vi "BASE_Reporting.vi"(8 "error in (no error)":errorcluster) -> (0 "error out":errorcluster)   [LabVIEW 2017]
uses:
  <vilib>/Utility/miscctls.llb/LVRangeTypeDef.ctl
  <vilib>/Utility/miscctls.llb/LVRowAndColumnTypeDef.ctl
  <vilib>/Utility/miscctls.llb/LVRowAndColumnUnsignedTypeDef.ctl
  <vilib>/addons/database/Connection.llb/DB Tools Open Connec (Path).vi
  <vilib>/Utility/file.llb/Write Delimited Spreadsheet (string).vi
  <vilib>/addons/database/NI_Database_API.lvlib
panel:
  in  "Machine Selection":string(combo)="ALL STATION"
  in  "Horizontal Slider Control":dbl(slide)=1.0 scale=0.0..19.0
  in  "Vertical Slider Control":dbl(slide)=1.0
  out "From Date":string
  out "appended path":path
  in  "SELECT FILTER":string(combo)="PART_NO"
  in  "Export to Excel":bool
  out "DESCRIPTION":string
  out "Data History Table":string[][](table)
  in  "TO DATE":timestamp format="%<%d/%m/%Y>T"
  in  "FROM DATE":timestamp format="%<%d/%m/%Y>T"
  in  "Back":bool
  in  "Show Report":bool
  # "BARCODE VERIFICATION SYSTEM REPORTS"
  # "Data History Table"
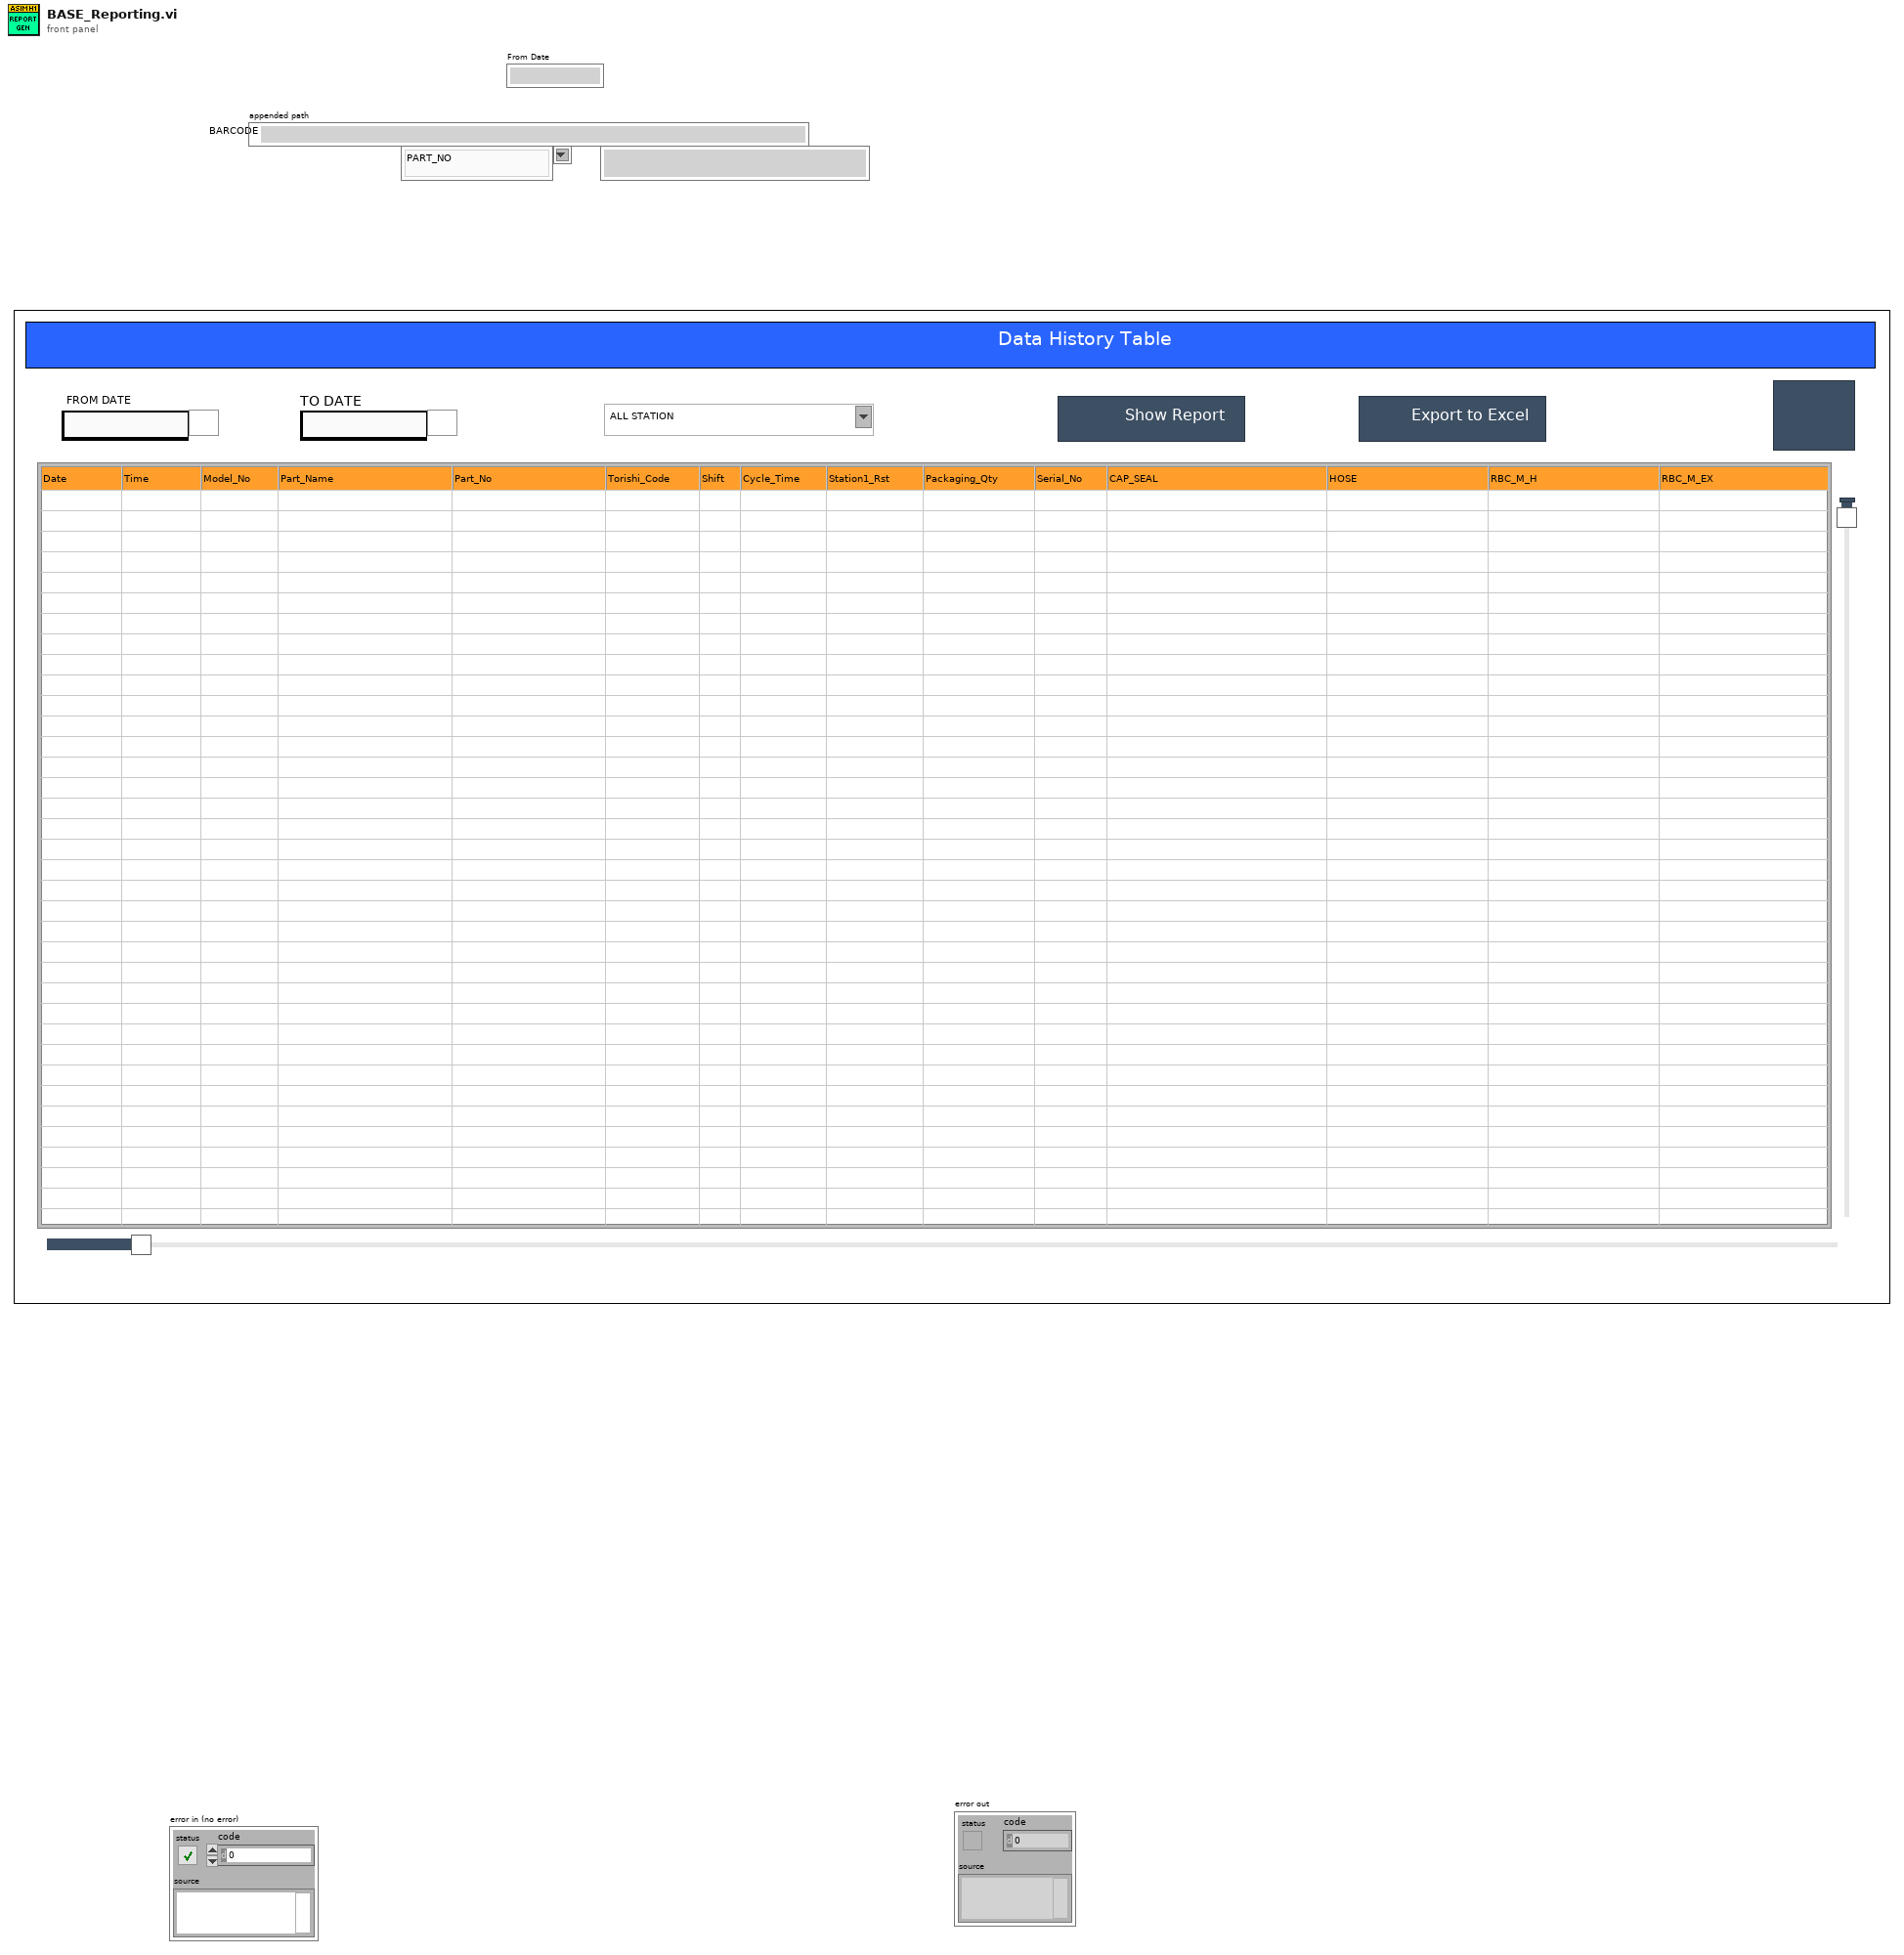
[diagram p1: front panel]
types:
  T1 = typedef "NI_Database_API.lvlib/Conn ObjectReference.ctl" = refnum<k1>
  T2 = typedef "LVRangeTypeDef.ctl" = cluster{"Minimum":dbl, "Maximum":dbl, "Increment":dbl, "Minor Increment":dbl, "Start":dbl}
  T3 = typedef "LVRowAndColumnTypeDef.ctl" = cluster{"Row":i32, "Column":i32}
  T4 = typedef "LVRowAndColumnUnsignedTypeDef.ctl" = cluster{"Row":u32, "Column":u32}
  T5 = enum32{"Invalid", "Standard", "Closed", "Hidden", "Minimized", "Maximized"}
  T6 = enum32{"invalid app kind", "Development System", "Run Time System", "Student Edition", "Embedded LabVIEW", "Evaluation", "Custom"}
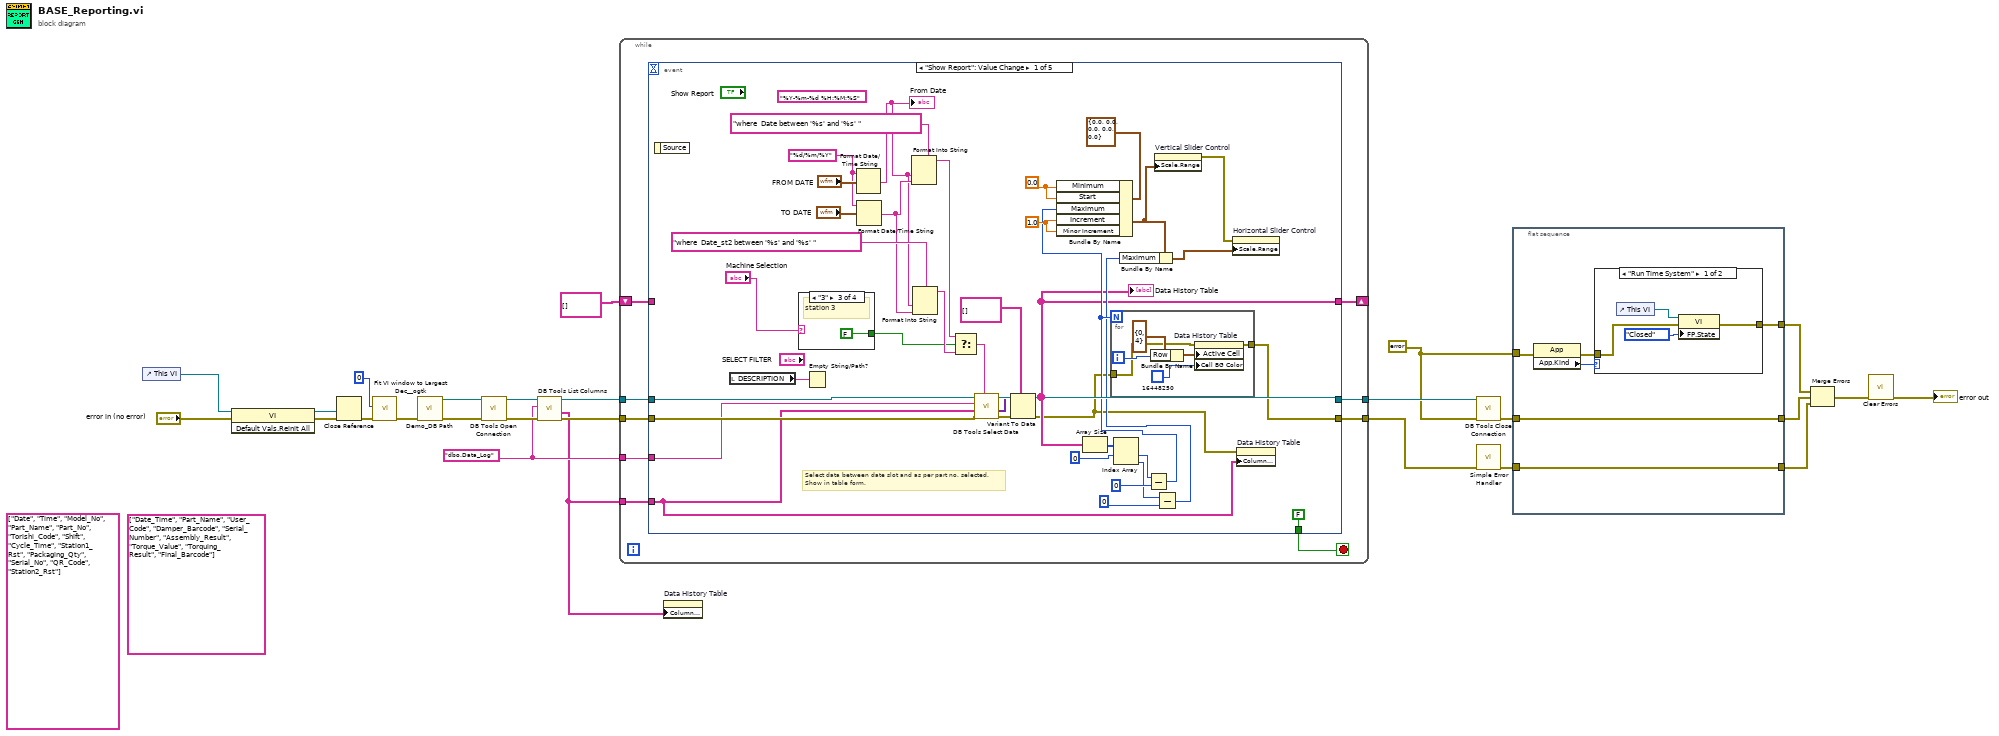
[diagram p0: block diagram]
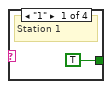
[diagram p3: hidden frame]
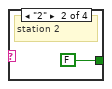
[diagram p4: hidden frame]
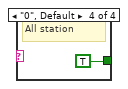
[diagram p5: hidden frame]
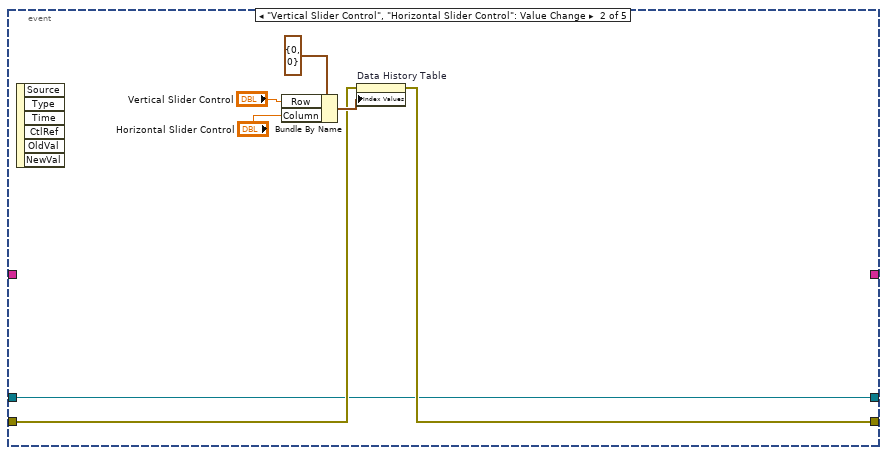
[diagram p6: hidden frame]
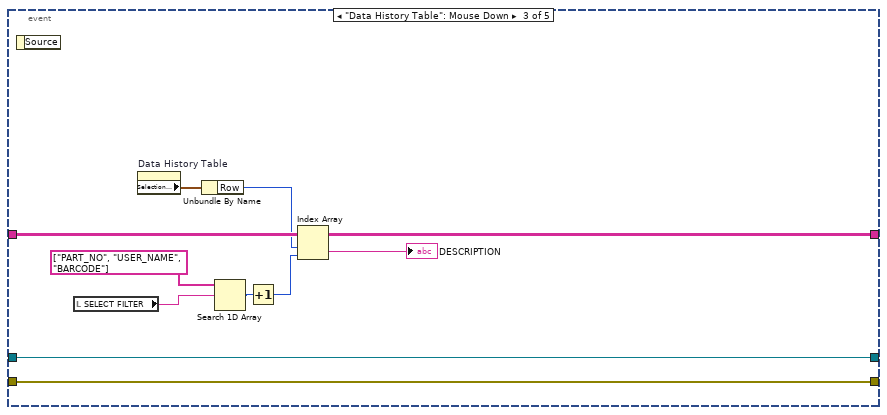
[diagram p7: hidden frame]
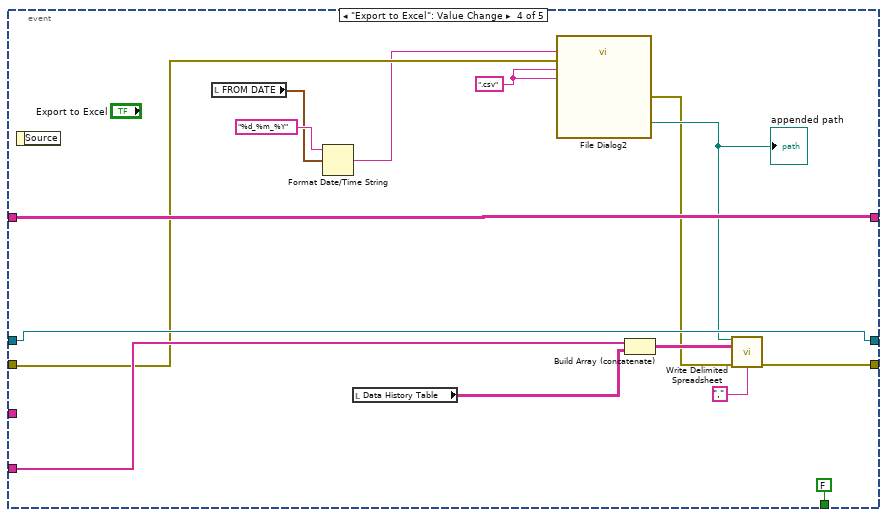
[diagram p8: hidden frame]
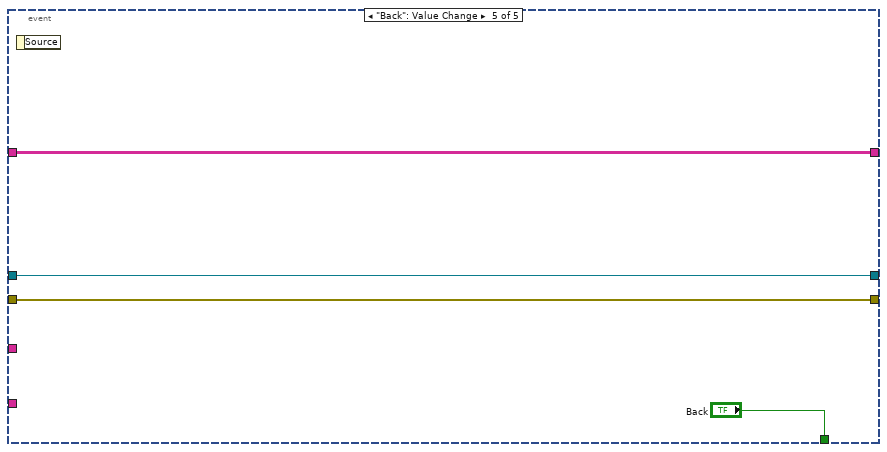
[diagram p9: hidden frame]
diagram:
  (unwired) string[] ["Date", "Time", "Model_No", "Part_Name", "Part_No", "Torishi_Code", "Shift", "Cycle_Time", "Station1_Rst", "Packaging_Qty", "Serial_No", "QR_Code", "Station2_Rst"] ("columns 2")
  w3 = "dbo.Data_Log" ("table")
  (unwired) string[] ["Date_Time", "Part_Name", "User_Code", "Damper_Barcode", "Serial_Number", "Assembly_Result", "Torque_Value", "Torquing_Result", "Final_Barcode"]
  w21 = errorcluster {"status"=FALSE, "code"=0, "source"=""} ("error in (no error)")
  n1 = control-ref of="This VI"() -> (w15:refnum<vi>)
  n2 = invoke class="VI" method="Default Vals.Reinit All"(reference=w15, error in="error in (no error)") -> (reference out=w13:refnum<vi>, error out=w12:errorcluster)  [unwired: 1 in, 1 out]
  n3 = Close Reference(reference=w13, error in (no error)=w12) -> (error out=w11:errorcluster)
  n4 = call <userlib>:"Fit VI window to Largest Dec__ogtk.vi"("error in (no error)"=w11, "border spacing (2 px)"=0) -> ("error out"=w4:errorcluster)  [unwired: 4 in, 1 out]
  n5 = call "Demo_DB Path.vi"("error in"=w4) -> ("error out"=w10:errorcluster, "DB Path"=w9:path)  [unwired: 9 in]
  n6 = call-poly <vilib>:"DB Tools Open Connection.vi"("error in (no error)"=w10, "connection information"=w9) -> ("error out"=w8:errorcluster, "connection reference"=w6:T1)  [unwired: 6 in]
  n7 = call <vilib>:"DB Tools List Columns.vi"("error in (no error)"=w8, "table"=w3, "connection reference"=w6) -> ("error out"=w7:errorcluster, "columns"=w2:string[], "connection reference out"=w5:T1)  [unwired: 1 in, 1 out]
  n8 = while {
    tunnel: w2 -> [w31]
    tunnel: w3 -> [w30]
    tunnel: w5 -> [w35]
    tunnel: [w32] -> w26
    tunnel: w7 -> [w34]
    tunnel: [w33] -> w24
    shift-right: [w28] -> _
    shift-left: string[][] [] -> [w27]
    stop <- w29 stop-if-true
    n9 = event shown="[0] \"Show Report\": Value Change" {
      selector: _ -> [_ _ _ _ _]
      dyn-events: _ -> [_ _ _ _ _]
      timeout: _ -> [_ _ _ _ _]
      tunnel: w35 -> [w74 w86 w98 w116 w119]
      tunnel: w34 -> [w73 w88 w97 w107 w118]
      tunnel: [w56 w87 w97 w111 w118] -> w33
      tunnel: [w72 w86 w98 w116 w119] -> w32
      tunnel: w31 -> [w42 _ _ w112 _]
      tunnel: w30 -> [w71 _ _ _ _]
      tunnel: [FALSE ("Back") _ _ FALSE ("Back") "Back"] -> w29
      tunnel: [w43 _ w101 w113 w117] -> w28
      tunnel: w27 -> [_ _ w101 w113 w117]
      event "Show Report": Value Change {
        w44 = 0.0 ("Start")
        w54 = 1.0 ("Increment")
        (unwired) "%Y-%m-%d %H:%M:%S"
        w61 = "%d/%m/%Y"
        # "Select data between date slot and as per part no. selected.\nShow in table form."
        n10 = event-data() -> ()  [unwired: 1 in, 1 out]
        n11 = local read "DESCRIPTION"() -> (w59:string)
        n12 = case shown="\"3\"" "Machine Selection" {
          tunnel: [TRUE FALSE FALSE TRUE] -> w36
          frame "1" {
            # "Station 1"
          }
          frame "2" {
            # "station 2"
          }
          frame "3" {
            # "station 3"
          }
          frame "0", Default {
            # "All station"
          }
        }
        n13 = Empty String/Path?(string/path=w59) -> ()  [unwired: 1 out]
        n14 = Format Date/Time String(time format string (%c)=w61, seconds (now)="FROM DATE") -> (date/time string=w38:string)  [unwired: 1 in]
        "From Date" <- w38
        n15 = Format Date/Time String(time format string (%c)=w61, seconds (now)="TO DATE") -> (date/time string=w39:string)  [unwired: 1 in]
        n16 = Format Into String(format string="where  Date between '%s' and '%s' ", w38, w39) -> (resulting string=w65:string)  [unwired: 2 in, 1 out]
        n17 = Format Into String(format string="where  Date_st2 between '%s' and '%s' ", w38, w39) -> (resulting string=w66:string)  [unwired: 2 in, 1 out]
        n18 = Select(t=w65, s=w36, f=w66) -> (s? t:f=w60:string)
        n19 = call <vilib>:"DB Tools Select Data.vi"("condition"=w60, "error in (no error)"=w73, "columns"=w42, "table"=w71, "connection reference"=w74) -> ("error out"=w67:errorcluster, "data"=w70:variant[][], "connection reference out"=w72:T1)  [unwired: 1 in]
        n20 = Variant To Data(error in=w67, type=string[][] [], Variant=w70) -> (data=w43:string[][], error out=w41:errorcluster)
        "Data History Table" <- w43
        n21 = Array Size(array=w43) -> (size(s)=w58:i32[])
        n22 = Index Array(array=w58, index #1=0 ("index")) -> (element #1=w49:i32, element #2=w46:i32)  [unwired: 1 in]
        n23 = Subtract(x=w49, y=0) -> (x-y=w48:i32)
        n24 = Bundle By Name(cluster=T2 {"Minimum"=0.0, "Maximum"=0.0, "Increment"=0.0, "Minor Increment"=0.0, "Start"=0.0} ("Scale.Range"), "Minimum"=w44, "Start"=w44, "Maximum"=w48, "Increment"=w54, "Minor Increment"=w54) -> (w53:T2)
        n25 = for {
          N: w48 -> [_]
          tunnel: w41 -> [w80]
          tunnel: [w79] -> w56
          i -> [w82]
          n26 = Bundle By Name(cluster=T3 {"Row"=0, "Column"=4} ("Active Cell:Active Cell"), "Row"=w82) -> (w83:T3)
          n27 = property on="Data History Table" class="Tbl (strict)"(error in=w80, "Active Cell"=w83, "Cell BG Color"=u32 16448250) -> (error out=w79:errorcluster)  [unwired: 1 in, 1 out]
        }
        n28 = property on="Vertical Slider Control" class="Slide (strict)"("Scale.Range"=w53) -> (error out=w51:errorcluster)  [unwired: 2 in, 1 out]
        n29 = Subtract(x=w46, y=0) -> (x-y=w47:i32)
        n30 = Bundle By Name(cluster=w53, "Maximum"=w47) -> (w52:T2)
        n31 = property on="Horizontal Slider Control" class="Slide (strict)"(error in=w51, "Scale.Range"=w52) -> ()  [unwired: 1 in, 2 out]
        n32 = property on="Data History Table" class="Tbl (strict)"(error in=w41, "Column Headers[]"=w42) -> ()  [unwired: 1 in, 2 out]
      }
      event "Vertical Slider Control", "Horizontal Slider Control": Value Change {
        n33 = event-data() -> ()  [unwired: 1 in, 6 out]
        n34 = Bundle By Name(cluster=T4 {"Row"=0, "Column"=0} ("Index Values"), "Row"="Vertical Slider Control", "Column"="Horizontal Slider Control") -> (w91:T4)
        n35 = property on="Data History Table" class="Tbl (strict)"(error in=w88, "Index Values"=w91) -> (error out=w87:errorcluster)  [unwired: 1 in, 1 out]
      }
      event "Data History Table": Mouse Down {
        n36 = event-data() -> ()  [unwired: 1 in, 1 out]
        n37 = local read "SELECT FILTER"() -> (w94:string)
        n38 = property on="Data History Table" class="Tbl (strict)"() -> ("Selection Start"=w100:T3)  [unwired: 2 in, 2 out]
        n39 = Unbundle By Name(w100) -> ("Row"=w99:i32)
        n40 = Search 1D Array(1D array=string[] ["PART_NO", "USER_NAME", "BARCODE"], element=w94) -> (index of element=w93:i32)  [unwired: 1 in]
        n41 = Increment(x=w93) -> (x+1=w92:i32)
        n42 = Index Array(array=w101, index (row)=w99, index (col)=w92) -> (element=→"DESCRIPTION":string)
      }
      event "Export to Excel": Value Change {
        w110 = ".csv" ("pattern label")
        n43 = event-data() -> ()  [unwired: 1 in, 1 out]
        n44 = local read "FROM DATE"() -> (w105:timestamp)
        n45 = Format Date/Time String(time format string (%c)="%d_%m_%Y", seconds (now)=w105) -> (date/time string=w104:string)  [unwired: 1 in]
        n46 = local read "Data History Table"() -> (w102:string[][])
        n47 = call "File Dialog2"("default name"=w104, "error in"=w107, "pattern (all files)"=w110, "pattern label"=w110) -> ("selected path"=w109:path, "error out"=w108:errorcluster)  [unwired: 8 in, 2 out]
        "appended path" <- w109
        n48 = Build Array (concatenate)(w112, w102) -> (w114:string[][])
        n49 = call-poly <vilib>:"Write Delimited Spreadsheet.vi"("file path (dialog if empty)"=w109, "2D data"=w114, "error in (no error)"=w108, "delimiter (\\t)"="," ("delimiter (\\t)")) -> ("error out"=w111:errorcluster)  [unwired: 10 in, 1 out]
      }
      event "Back": Value Change {
        n50 = event-data() -> ()  [unwired: 1 in, 1 out]
      }
    }
  }
  n51 = property on="Data History Table" class="Tbl (strict)"("Column Headers[]"=w2) -> ()  [unwired: 2 in, 2 out]
  n52 = call <vilib>:"DB Tools Close Connection.vi"("error in (no error)"=w21, "connection reference"=w26) -> ("error out"=w19:errorcluster)  [unwired: 5 in]
  n53 = call <vilib>:"Simple Error Handler.vi"("error in (no error)"=w24) -> ("error out"=w17:errorcluster)  [unwired: 4 in, 4 out]
  n54 = flat-sequence {
    tunnel: [w124] -> w22
    tunnel: w21 -> [w123]
    tunnel: [w122] -> w20
    tunnel: w19 -> [w122]
    tunnel: [w121] -> w18
    tunnel: w17 -> [w121]
    frame #0 {
      n55 = property class="App"(error in=w123) -> (error out=w125:errorcluster, "App.Kind"=w126:T6)  [unwired: 1 in, 1 out]
      n56 = case shown="\"Run Time System\"" w126 {
        tunnel: w125 -> [w128 w131]
        tunnel: [w127 w131] -> w124
        frame "Run Time System" {
          n57 = control-ref of="This VI"() -> (w130:refnum<vi>)
          n58 = property class="VI"(reference=w130, error in=w128, "FP.State"=T5."Closed" ("Front Panel Window:State")) -> (error out=w127:errorcluster)  [unwired: 1 out]
        }
        frame "Development System", Default {
        }
      }
    }
  }
  n59 = Merge Errors(w22, w20, w18) -> (w23:errorcluster)
  n60 = call <vilib>:"Clear Errors.vi"("error in (no error)"=w23) -> ("error out"=→"error out":errorcluster)  [unwired: 5 in, 1 out]
